vi "J1939 Network Address Lookup Table.vi"(7 "Action":T2, 8 "error in (no error)":errorcluster, 9 "Address":u8, 10 "Data":T1 {"Name" format="%.0x"}, 11 "ref in":T3) -> (0 "error out":errorcluster {"code" min=0 max=0}, 1 "Found?":bool, 2 "Data":T1 {"Name" format="%.0x"}, 4 "All Data":T1[](array[typedef]) {"Name" format="%.0x"})   [LabVIEW 2013, in "J1939.lvlib"]
uses:
  J1939.lvlib
  J1939 Address Table Reference.ctl
  J1939 Address Lookup Table Data.ctl
  J1939 Address Lookup Table Action.ctl
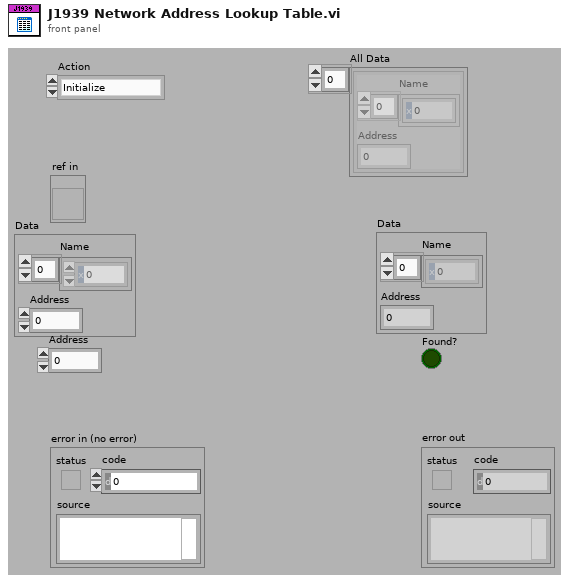
[diagram p1: front panel]
types:
  T1 = typedef "J1939.lvlib/J1939 Address Lookup Table Data.ctl" = cluster{"Name":u8[], "Address":u8}
  T2 = typedef "J1939.lvlib/J1939 Address Lookup Table Action.ctl" = enum16{"Initialize", "Add", "Get", "Remove", "Get All"}
  T3 = typedef "J1939.lvlib/J1939 Address Table Reference.ctl" = refnum<vi>
  T4 = typedef "J1939 Addresses Table Data.ctl" = cluster{"Name":u8[], "Address":u8}
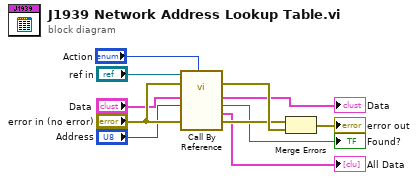
[diagram p0: block diagram]
diagram:
  n1 = call-by-ref "?"(reference="ref in", error in="error in (no error)", "Action"="Action", 8:"error in (no error)"="error in (no error)", "Address"="Address", "Data"="Data") -> (error out=w10:errorcluster, 0:"error out"=w7:errorcluster, "All Data"=→"All Data":T4[], "Found?"=→"Found?":bool, "Data"=→"Data":T4)  [unwired: 4 in, 1 out]
  n2 = Merge Errors(w7, w10) -> (→"error out":errorcluster)
